vi "Begin.vi"(11 "Image Size":T2=enum."320x240") -> (0 "error out":errorcluster)   [LabVIEW 2011]
doc: "Called before other user functions, this VI is expected to open initial I/O refnums, load in file data, and do all program initialization. Notice that the <B>error out</B> terminal is simply used for data flow. Wiring it to other structures or subVIs ensures that this VI runs first."
uses:
  <vilib>/Rock Robotics/WPI/Camera/WPI_CameraImageSize.ctl
  <vilib>/Rock Robotics/WPI/Encoder/WPI_EncoderType.ctl
  <vilib>/Rock Robotics/SystemInterfaces/DIO/FPGA_DIOPWMChannel.ctl
  <vilib>/Rock Robotics/WPI/Joystick/WPI_JoystickDeviceEnum.ctl
  <vilib>/Rock Robotics/SystemInterfaces/Typedef/FPGA_TypedefDigitalModule.ctl
  <vilib>/Rock Robotics/SystemInterfaces/DIO/FPGA_DIOChannel.ctl
  <vilib>/Rock Robotics/WPI/SafetyOutput/WPI_SafetyOutputConfigMenu.ctl
  <vilib>/Rock Robotics/WPI/Solenoid/WPI_SolenoidChannel.ctl
  <vilib>/Rock Robotics/SystemInterfaces/DIO/FPGA_DIORelayChannel.ctl
  <vilib>/Rock Robotics/SystemInterfaces/Typedef/FPGA_TypedefSolenoidModule.ctl
  <vilib>/Rock Robotics/WPI/MotorControl/WPI_MotorControlOpen Victor.vi
  <vilib>/Rock Robotics/WPI/Counter/WPI_CounterDigitalInputToDigitalSource.vi
  <vilib>/Rock Robotics/WPI/Solenoid/WPI_SolenoidOpenSingle.vi
  <vilib>/Rock Robotics/WPI/Solenoid/WPI_SolenoidOpenDouble.vi
  <vilib>/Rock Robotics/WPI/Compressor/WPI_CompressorGetSetRefNum.vi
  <vilib>/Rock Robotics/WPI/Camera/WPI_CameraWhite Balance Values.ctl
  <vilib>/Rock Robotics/WPI/Camera/WPI_CameraExposure Values.ctl
  <vilib>/Rock Robotics/WPI/Camera/WPI_CameraFrameRate.ctl
panel:
  in  "Invert Direction Right":bool
  in  "Decoding Type Right":T1=enum."4x"
  in  "DistancePerCount Right":dbl=0.06731984257692414
  in  "Minimum Rate Right":dbl=20.0
  in  "Number Samples to Average Right":u8=1 min=1 max=128
  in  "Number Samples to Average Left":u8=1 min=1 max=128
  in  "Minimum Rate Left":dbl=20.0
  in  "DistancePerCount Left":dbl=0.06731984257692414
  in  "Decoding Type Left":T1=enum."4x"
  in  "Invert Direction Left":bool=TRUE
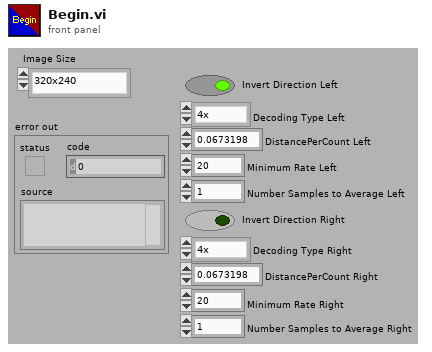
[diagram p1: front panel]
types:
  T1 = typedef "WPI_EncoderType.ctl" = enum16{"1x", "2x", "4x"}
  T2 = typedef "WPI_CameraImageSize.ctl" = enum16{"640x480", "320x240", "160x120"}
  T3 = typedef "WPI_SolenoidChannel.ctl" = enum8{"Solenoid 1", "Solenoid 2", "Solenoid 3", "Solenoid 4", "Solenoid 5", "Solenoid 6", "Solenoid 7", "Solenoid 8", "Invalid"}
  T4 = typedef "FPGA_TypedefSolenoidModule.ctl" = enum16{"Solenoid Module 1", "Solenoid Module 2"}
  T5 = typedef "FPGA_DIORelayChannel.ctl" = enum8{"Relay 1", "Relay 2", "Relay 3", "Relay 4", "Relay 5", "Relay 6", "Relay 7", "Relay 8", "Invalid"}
  T6 = typedef "FPGA_TypedefDigitalModule.ctl" = enum16{"Digital Module 1", "Digital Module 2"}
  T7 = typedef "FPGA_DIOChannel.ctl" = enum8{"DIO 1", "DIO 2", "DIO 3", "DIO 4", "DIO 5", "DIO 6", "DIO 7", "DIO 8", "DIO 9", "DIO 10", "DIO 11", "DIO 12", "DIO 13", "DIO 14", "Invalid"}
  T8 = typedef "WPI_SafetyOutputConfigMenu.ctl" = enum16{"Enable", "Disable"}
  T9 = typedef "FPGA_DIOPWMChannel.ctl" = enum8{"PWM 1", "PWM 2", "PWM 3", "PWM 4", "PWM 5", "PWM 6", "PWM 7", "PWM 8", "PWM 9", "PWM 10", "Invalid"}
  T10 = typedef "WPI_JoystickDeviceEnum.ctl" = enum16{"USB 1", "USB 2", "USB 3", "USB 4", "Kinect 1", "Kinect 2"}
  T11 = typedef "WPI_DigitalInputDevRef.ctl" = cluster{"DevStatus":errorcluster, "DIO Channel":T7, "Digital Module":T6}
  T12 = typedef "WPI_MotorControlDeviceRef.ctl" = cluster{"DeviceStatus":errorcluster, "Type":enum16{"PWM", "CAN"}, "PWM":cluster{"Digital Module":T6, "PWM Channel":T9, "DeadBand":T13}, "CAN":cluster{"Device Number":u8, "Control Mode":T14, "Semaphore":T15, "Max Vout":dbl}, "Invert":bool, "TransformRef":T16, "InvTransformRef":T16}
  T13 = typedef "WPI_PWMDeadband.ctl" = cluster{"Name":string, "maxPositivePwm":i32, "minPositivePwm":i32, "centerPwm":i32, "maxNegativePwm":i32, "minNegativePwm":i32, "angularRange":u16}
  T14 = typedef "WPI_CANJaguar_ControlMode.ctl" = enum8{"Percent VBus", "Current", "Speed", "Position", "Voltage"}
  T15 = typedef "Semaphore RefNum" = refnum<k1>
  T16 = typedef "WPI_PWMTransform_ConPane.ctl" = refnum<vi>
  T17 = typedef "WPI_JoystickDevRef.ctl" = cluster{"Device":T10}
  T18 = typedef "WPI_RobotDriveDevRef.ctl" = cluster{"DevStatus":errorcluster, "Motors[]":T12[], "Square Inputs":bool, "Max Output":dbl, "Isochronous":bool}
  T19 = typedef "FPGA_CounterEncoderSourceConvertionLVSourceType.ctl" = cluster{"DevStatus":errorcluster, "AnalogTriggerMode?":bool, "DigitalMode":cluster{"Digital Module":T6, "DIO Channel":T20}, "AnalogTriggerMode":cluster{"AnalogTriggerIndex":T21, "OutputType":T22}}
  T20 = typedef "FPGA_DIODigitalSourceChannel.ctl" = enum8{"DIO 1", "DIO 2", "DIO 3", "DIO 4", "DIO 5", "DIO 6", "DIO 7", "DIO 8", "DIO 9", "DIO 10", "DIO 11", "DIO 12", "DIO 13", "DIO 14", "Disabled"}
  T21 = typedef "FPGA_AnalogTriggerIndex.ctl" = enum8{"Trig 0", "Trig 1", "Trig 2", "Trig 3", "Trig 4", "Trig 5", "Trig 6", "Trig 7", "Invalid"}
  T22 = typedef "FPGA_AnalogTriggerOutType.ctl" = enum16{"InWindow", "TriggerState", "Rising", "Falling"}
  T23 = typedef "WPI_EncoderDevRef.ctl" = cluster{"DevStatus":errorcluster, "EncoderIndex":T24, "CounterIndex":T25, "DistancePerCount":dbl, "Decoding Type":T1}
  T24 = typedef "FPGA_EncoderIdx.ctl" = enum8{"Enc 0", "Enc 1", "Enc 2", "Enc 3", "Invalid"}
  T25 = typedef "FPGA_CounterCtrSystemIndex.ctl" = enum8{"Ctr 0", "Ctr 1", "Ctr 2", "Ctr 3", "Ctr 4", "Ctr 5", "Ctr 6", "Ctr 7", "Invalid"}
  T26 = typedef "WPI_CameraFrameRate.ctl" = u32
  T27 = typedef "WPI_CameraExposure Values.ctl" = enum16{"Auto", "Flicker-free 50 Hz", "Flicker-free 60 Hz", "Hold current"}
  T28 = typedef "WPI_CameraWhite Balance Values.ctl" = enum16{"Auto", "Fixed indoor", "Fixed outdoor 1", "Fixed outdoor 2", "Fixed fluorescent 1", "Fixed fluorescent 2", "Hold current"}
  T29 = typedef "WPI_CameraDevRef.ctl" = cluster{"Camera Address":string, "CameraStatus":errorcluster, "Acquire Image Notifier":refnum<notifier>}
  T30 = typedef "WPI_SolenoidDevRef.ctl" = cluster{"DevStatus":errorcluster, "Solenoid Module":T4, "Forward Solenoid Channel":T3, "Reverse Solenoid Channel":T3}
  T31 = typedef "WPI_CompressorDevRef.ctl" = cluster{"DevStatus":errorcluster, "DigitalInputDevRef":T11, "RelayDevRef":T32}
  T32 = typedef "WPI_RelayDevRef.ctl" = cluster{"DevStatus":errorcluster, "Relay Channel":T5, "Digital Module":T6, "Relay Direction":T33}
  T33 = typedef "WPI_RelayDirection.ctl" = enum16{"Both directions", "Forward only", "Reverse only"}
  T34 = typedef "WPI_ServoDeviceRef.ctl" = cluster{"DeviceStatus":errorcluster, "Digital Module":T6, "PWM Channel":T9, "DeadBand":T13}
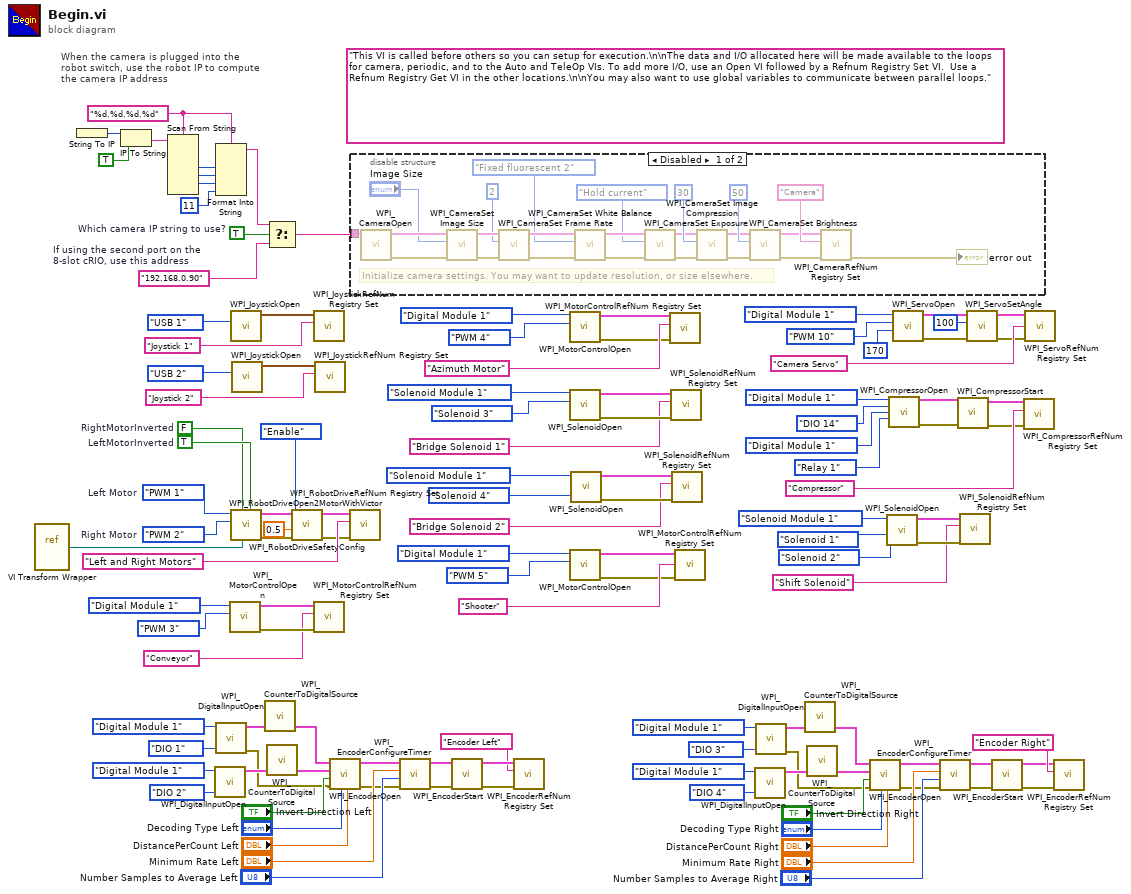
[diagram p0: block diagram]
diagram:
  w104 = TRUE  # Which camera IP string to use?
  w108 = "%d.%d.%d.%d" ("format string")
  (unwired) "This VI is called before others so you can setup for execution.\n\nThe data and I/O allocated here will be made available to the loops for camera, periodic, and to the Auto and TeleOp VIs. To add more I/O, use an Open VI followed by a Refnum Registry Set VI.  Use a Refnum Registry Get VI in the other locations.\n\nYou may also want to use global variables to communicate between parallel loops."
  w117 = FPGA_DIOPWMChannel."PWM 2"  # Right Motor
  w118 = FPGA_DIOPWMChannel."PWM 1"  # Left Motor
  w105 = "192.168.0.90"  # If using the second port on the 8-slot cRIO, use this address
  w103 = TRUE  # LeftMotorInverted
  w102 = FALSE  # RightMotorInverted
  # "When the camera is plugged into the\nrobot switch, use the robot IP to compute\nthe camera IP address"
  n1 = vi-ref "VI Transform Wrapper.vi"() -> (w37:refnum<vi>)
  n2 = String To IP() -> (0:w115:u32)  [unwired: 1 in]
  n3 = IP To String(1:TRUE ("dot notation? (F)"), 2:w115) -> (0:w113:string)
  n4 = Scan From String(format string=w108, input string=w113) -> (output 1=w112:i32, output 2=w111:i32, output 3=w110:i32)  [unwired: 7 in, 3 out]
  n5 = call <vilib>:"WPI_DigitalInputOpen.vi"("DIO Channel"=FPGA_DIOChannel."DIO 2", "Digital Module (Module 1)"=FPGA_TypedefDigitalModule."Digital Module 1") -> ("DigitalInputDevRef"=w79:T11)  [unwired: 1 in, 8 out]
  n6 = Format Into String(format string=w108, w112, w111, w110, 11 ("Compression")) -> (resulting string=w106:string)  [unwired: 2 in, 1 out]
  n7 = call <vilib>:"WPI_DigitalInputOpen.vi"("DIO Channel"=FPGA_DIOChannel."DIO 1", "Digital Module (Module 1)"=FPGA_TypedefDigitalModule."Digital Module 1") -> ("error out"=w39:errorcluster, "DigitalInputDevRef"=w78:T11)  [unwired: 1 in, 7 out]
  n8 = call-poly <vilib>:"WPI_MotorControlOpen.vi"("PWM Channel"=FPGA_DIOPWMChannel."PWM 3", "Digital Module (Module 1)"=FPGA_TypedefDigitalModule."Digital Module 1") -> ("error out"=w86:errorcluster, "MotorControlDeviceRef"=w88:T12)  [unwired: 8 in]
  n9 = call <vilib>:"WPI_JoystickOpen.vi"("JoystickDevice"=WPI_JoystickDeviceEnum."USB 1") -> ("JoystickDevRef"=w120:T17)  [unwired: 10 out]
  n10 = call "WPI_RobotDriveOpen2MotorWithVictor.vi"("Right Motor Inverted"=w103, "TransformVIRef"=w37, "Left Motor Inverted"=w102, "Right Motor"=w117, "Left Motor"=w118) -> ("error out"=w36:errorcluster, "RobotDriveDevRef"=w34:T18)  [unwired: 5 in]
  n11 = call <vilib>:"WPI_JoystickOpen.vi"("JoystickDevice"=WPI_JoystickDeviceEnum."USB 2") -> ("JoystickDevRef"=w100:T17)  [unwired: 10 in]
  n12 = call-poly <vilib>:"WPI_CounterToDigitalSource.vi"("DigitalInputDevRef"=w78) -> ("Digital Source"=w77:T19)  [unwired: 6 out]
  n13 = Select(t=w106, s=w104, f=w105) -> (s? t:f=w107:string)
  n14 = call-poly <vilib>:"WPI_CounterToDigitalSource.vi"("DigitalInputDevRef"=w79) -> ("Digital Source"=w76:T19)  [unwired: 6 out]
  n15 = call <vilib>:"WPI_RobotDriveSafetyConfig.vi"("error in (no error)"=w36, "timeout (s)"=0.5, "mode"=WPI_SafetyOutputConfigMenu."Enable", "RobotDriveDevRef"=w34) -> ("error out"=w35:errorcluster, "RobotDriveDevRef"=w33:T18)  [unwired: 6 in]
  n16 = call <vilib>:"WPI_JoystickRefNum Registry Set.vi"("refnum name"="Joystick 1", "JoystickDevRef"=w120) -> ()  [unwired: 1 in, 9 out]
  n17 = call <vilib>:"WPI_MotorControlRefNum Registry Set.vi"("error in (no error)"=w86, "refnum name"="Conveyor", "MotorControlDevRef"=w88) -> ()  [unwired: 7 in, 2 out]
  n18 = call <vilib>:"WPI_JoystickRefNum Registry Set.vi"("refnum name"="Joystick 2", "JoystickDevRef"=w100) -> ()  [unwired: 8 in, 2 out]
  n19 = call <vilib>:"WPI_EncoderOpen.vi"("DistancePerCount"="DistancePerCount Left", "Decoding Type"="Decoding Type Left", "error in (no error)"=w39, "Invert Direction (False)"="Invert Direction Left", "BSource"=w76, "ASource"=w77) -> ("error out"=w40:errorcluster, "EncoderDevRef"=w75:T23)  [unwired: 2 in, 2 out]
  n20 = call <vilib>:"WPI_RobotDriveRefNum Registry Set.vi"("error in (no error)"=w35, "refnum name"="Left and Right Motors", "RobotDriveDevRef"=w33) -> ()  [unwired: 9 out]
  n21 = disable-structure shown="Disabled" {
    disable-tunnel: w107 -> [w123 _]
    frame Disabled {
      # "Initialize camera settings. You may want to update resolution, or size elsewhere."
      n22 = call <vilib>:"WPI_CameraOpen.vi"("Camera Address"=w123) -> ("error out"=w135:errorcluster, "CameraDevRef"=w136:T29)  [unwired: 1 in, 8 out]
      n23 = call <vilib>:"WPI_CameraSet Image Size.vi"("error in (no error)"=w135, "Image Size"="Image Size", "CameraDevRef"=w136) -> ("error out"=w134:errorcluster, "CameraDevRef Out"=w137:T29)  [unwired: 7 out]
      n24 = call <vilib>:"WPI_CameraSet Frame Rate.vi"("error in (no error)"=w134, "Frame Rate (fps)"=T26 2, "CameraDevRef"=w137) -> ("error out"=w133:errorcluster, "CameraDevRef Out"=w139:T29)  [unwired: 7 out]
      n25 = call <vilib>:"WPI_CameraSet White Balance.vi"("error in (no error)"=w133, "White Balance"=WPI_CameraWhite_Balance_Values."Fixed fluorescent 2", "CameraDevRef"=w139) -> ("error out"=w132:errorcluster, "CameraDevRef Out"=w138:T29)  [unwired: 7 out]
      n26 = call <vilib>:"WPI_CameraSet Exposure.vi"("error in (no error)"=w132, "Exposure"=WPI_CameraExposure_Values."Hold current", "CameraDevRef"=w138) -> ("error out"=w131:errorcluster, "CameraDevRef Out"=w141:T29)  [unwired: 7 out]
      n27 = call <vilib>:"WPI_CameraSet Image Compression.vi"("error in (no error)"=w131, "Compression"=30, "CameraDevRef"=w141) -> ("error out"=w130:errorcluster, "CameraDevRef Out"=w140:T29)  [unwired: 7 out]
      n28 = call <vilib>:"WPI_CameraSet Brightness.vi"("error in (no error)"=w130, "Brightness"=50, "CameraDevRef"=w140) -> ("error out"=w128:errorcluster, "CameraDevRef Out"=w129:T29)  [unwired: 7 out]
      n29 = call <vilib>:"WPI_CameraRefNum Registry Set.vi"("error in (no error)"=w128, "refnum name"="Camera", "CameraDevRef"=w129) -> ("error out"=→"error out":errorcluster)  [unwired: 8 out]
    }
    frame Enabled {
    }
  }
  n30 = call <vilib>:"WPI_EncoderConfigureTimer.vi"("error in (no error)"=w40, "Number Samples to Average"="Number Samples to Average Left", "Minimum Rate"="Minimum Rate Left", "EncoderDevRef"=w75) -> ("error out"=w43:errorcluster, "EncoderDevRef"=w74:T23)  [unwired: 6 out]
  n31 = call <vilib>:"WPI_EncoderStart.vi"("error in (no error)"=w43, "EncoderDevRef"=w74) -> ("error out"=w68:errorcluster, "EncoderDevRef"=w67:T23)  [unwired: 8 out]
  n32 = call <vilib>:"WPI_EncoderRefNum Registry Set.vi"("error in (no error)"=w68, "refnum name"="Encoder Left", "EncoderDevRef"=w67) -> ()  [unwired: 7 in, 2 out]
  n33 = call-poly <vilib>:"WPI_MotorControlOpen.vi"("PWM Channel"=FPGA_DIOPWMChannel."PWM 4", "Digital Module (Module 1)"=FPGA_TypedefDigitalModule."Digital Module 1") -> ("error out"=w95:errorcluster, "MotorControlDeviceRef"=w97:T12)  [unwired: 8 in]
  n34 = call-poly <vilib>:"WPI_SolenoidOpen.vi"("Solenoid Channel"=WPI_SolenoidChannel."Solenoid 3", "Solenoid Module (Module 1)"=FPGA_TypedefSolenoidModule."Solenoid Module 1") -> ("error out"=w8:errorcluster, "SolenoidDevRef"=w9:T30)  [unwired: 1 in, 7 out]
  n35 = call-poly <vilib>:"WPI_MotorControlOpen.vi"("PWM Channel"=FPGA_DIOPWMChannel."PWM 5", "Digital Module (Module 1)"=FPGA_TypedefDigitalModule."Digital Module 1") -> ("error out"=w87:errorcluster, "MotorControlDeviceRef"=w92:T12)  [unwired: 8 in]
  n36 = call-poly <vilib>:"WPI_SolenoidOpen.vi"("Solenoid Channel"=WPI_SolenoidChannel."Solenoid 4", "Solenoid Module (Module 1)"=FPGA_TypedefSolenoidModule."Solenoid Module 1") -> ("error out"=w5:errorcluster, "SolenoidDevRef"=w6:T30)  [unwired: 1 in, 7 out]
  n37 = call <vilib>:"WPI_MotorControlRefNum Registry Set.vi"("error in (no error)"=w95, "refnum name"="Azimuth Motor", "MotorControlDevRef"=w97) -> ()  [unwired: 7 in, 2 out]
  n38 = call <vilib>:"WPI_SolenoidRefNum Registry Set.vi"("error in (no error)"=w8, "refnum name"="Bridge Solenoid 1", "SolenoidDevRef"=w9) -> ()  [unwired: 7 in, 2 out]
  n39 = call <vilib>:"WPI_SolenoidRefNum Registry Set.vi"("error in (no error)"=w5, "refnum name"="Bridge Solenoid 2", "SolenoidDevRef"=w6) -> ()  [unwired: 7 in, 2 out]
  n40 = call <vilib>:"WPI_MotorControlRefNum Registry Set.vi"("error in (no error)"=w87, "refnum name"="Shooter", "MotorControlDevRef"=w92) -> ()  [unwired: 7 in, 2 out]
  n41 = call <vilib>:"WPI_DigitalInputOpen.vi"("DIO Channel"=FPGA_DIOChannel."DIO 4", "Digital Module (Module 1)"=FPGA_TypedefDigitalModule."Digital Module 1") -> ("DigitalInputDevRef"=w52:T11)  [unwired: 1 in, 8 out]
  n42 = call <vilib>:"WPI_DigitalInputOpen.vi"("DIO Channel"=FPGA_DIOChannel."DIO 3", "Digital Module (Module 1)"=FPGA_TypedefDigitalModule."Digital Module 1") -> ("error out"=w38:errorcluster, "DigitalInputDevRef"=w53:T11)  [unwired: 1 in, 7 out]
  n43 = call-poly <vilib>:"WPI_CounterToDigitalSource.vi"("DigitalInputDevRef"=w53) -> ("Digital Source"=w54:T19)  [unwired: 6 out]
  n44 = call-poly <vilib>:"WPI_CounterToDigitalSource.vi"("DigitalInputDevRef"=w52) -> ("Digital Source"=w55:T19)  [unwired: 6 out]
  n45 = call <vilib>:"WPI_EncoderOpen.vi"("DistancePerCount"="DistancePerCount Right", "Decoding Type"="Decoding Type Right", "error in (no error)"=w38, "Invert Direction (False)"="Invert Direction Right", "BSource"=w55, "ASource"=w54) -> ("error out"=w41:errorcluster, "EncoderDevRef"=w56:T23)  [unwired: 2 in, 2 out]
  n46 = call-poly <vilib>:"WPI_SolenoidOpen.vi"("Reverse Solenoid Channel"=WPI_SolenoidChannel."Solenoid 2", "Forward Solenoid Channel"=WPI_SolenoidChannel."Solenoid 1" ("Solenoid Channel"), "Solenoid Module (Module 1)"=FPGA_TypedefSolenoidModule."Solenoid Module 1") -> ("error out"=w25:errorcluster, "SolenoidDevRef"=w24:T30)  [unwired: 1 in, 6 out]
  n47 = call <vilib>:"WPI_CompressorOpen.vi"("Pressure Switch Digital Module (Module 1)"=FPGA_TypedefDigitalModule."Digital Module 1", "Pressure Switch DIO Channel"=FPGA_DIOChannel."DIO 14", "Relay Digital Module (Module 1)"=FPGA_TypedefDigitalModule."Digital Module 1", "Relay Channel"=FPGA_DIORelayChannel."Relay 1") -> ("CompressorDevRef"=w16:T31, "error out"=w14:errorcluster)  [unwired: 1 in, 9 out]
  n48 = call <vilib>:"WPI_ServoOpen.vi"("Angular Range"=u16 170, "PWM Channel"=FPGA_DIOPWMChannel."PWM 10", "Digital Module (Module 1)"=FPGA_TypedefDigitalModule."Digital Module 1") -> ("error out"=w29:errorcluster, "ServoDeviceRef"=w30:T34)  [unwired: 7 in]
  n49 = call <vilib>:"WPI_EncoderConfigureTimer.vi"("error in (no error)"=w41, "Number Samples to Average"="Number Samples to Average Right", "Minimum Rate"="Minimum Rate Right", "EncoderDevRef"=w56) -> ("error out"=w42:errorcluster, "EncoderDevRef"=w57:T23)  [unwired: 6 out]
  n50 = call <vilib>:"WPI_CompressorStart.vi"("error in (no error)"=w14, "CompressorDevRef"=w16) -> ("error out"=w13:errorcluster, "CompressorDevRef"=w15:T31)  [unwired: 8 in]
  n51 = call <vilib>:"WPI_SolenoidRefNum Registry Set.vi"("error in (no error)"=w25, "refnum name"="Shift Solenoid", "SolenoidDevRef"=w24) -> ()  [unwired: 7 in, 2 out]
  n52 = call <vilib>:"WPI_ServoSetAngle.vi"("error in (no error)"=w29, "Angle"=100, "ServoDeviceRef"=w30) -> ("error out"=w27:errorcluster, "ServoDeviceRef"=w28:T34)  [unwired: 7 in]
  n53 = call <vilib>:"WPI_EncoderStart.vi"("error in (no error)"=w42, "EncoderDevRef"=w57) -> ("error out"=w63:errorcluster, "EncoderDevRef"=w64:T23)  [unwired: 8 out]
  n54 = call <vilib>:"WPI_CompressorRefNum Registry Set.vi"("error in (no error)"=w13, "refnum name"="Compressor", "CompressorDevRef"=w15) -> ()  [unwired: 7 in, 2 out]
  n55 = call <vilib>:"WPI_ServoRefNum Registry Set.vi"("error in (no error)"=w27, "refnum name"="Camera Servo", "ServoDeviceRef"=w28) -> ()  [unwired: 7 in, 2 out]
  n56 = call <vilib>:"WPI_EncoderRefNum Registry Set.vi"("error in (no error)"=w63, "refnum name"="Encoder Right", "EncoderDevRef"=w64) -> ()  [unwired: 7 in, 2 out]
